vi "OpenCVCam_CastUIEvent.vi"(11 "UIEvent":T2) -> (1 "Data":variant, 2 "ApplicationGUI out":refnum<class "OpenCVCam.lvclass">, 3 "UiEventNames":T1)   [LabVIEW 2021, in "OpenCVCam.lvclass"]
uses:
  OpenCVCam.lvclass
  OpenCVCam_UiCallBackEvents.ctl
  OpenCVCam.lvclass/OpenCVCam.ctl
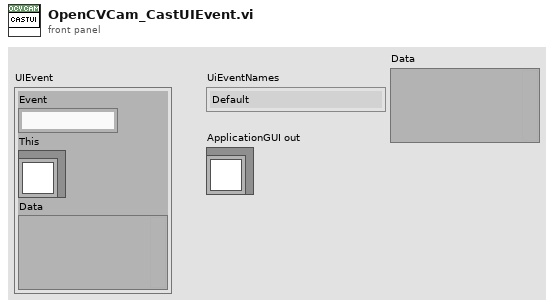
[diagram p1: front panel]
types:
  T1 = typedef "OpenCVCam.lvclass/OpenCVCam_UiCallBackEvents.ctl" = enum16{"Default", "PersistentDataUpdated", "NewPicture", "Worker 1: Do Something"}
  T2 = cluster{"Event":string, "This":refnum<class>, "Data":variant}
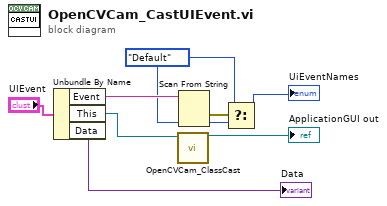
[diagram p0: block diagram]
diagram:
  w2 = OpenCVCam_UiCallBackEvents."Default" ("UiEventNames")
  n1 = Unbundle By Name("UIEvent") -> ("Event"=w7:string, "This"=w6:refnum<class>, "Data"=→"Data":variant)
  n2 = call "OpenCVCam_ClassCast.vi"("OpenCVCam in"=w6) -> ("OpenCVCam out"=→"ApplicationGUI out":refnum<class "OpenCVCam.lvclass">)  [unwired: 10 in]
  n3 = Scan From String(input string=w7, default 1=w2) -> (error out=w5:errorcluster, output 1=w4:T1)  [unwired: 3 in, 2 out]
  n4 = Select(t=w2, s=w5, f=w4) -> (s? t:f=→"UiEventNames":T1)
